vi "oa_SCL Draw XY Data.vi"(4 "[sized scatter plot cosmetics]":T1={"min size"=1, "max size"=5, "maps to max size"=5, "color array"=[16776960, 65280, 16711680, 255]}, 6 "xy cosmetics":T3={"plot color"=16776960, "plot type"=enum."connected points", "baseline"=0.0} {"baseline" format="%0.2f"}, 8 "xy data":cluster{"x":dbl, "y":dbl}[](array[cluster]) {"y" format="%0.2f"; "x" format="%0.2f"}, 9 "y scale factors":cluster{"a":dbl, "b":dbl, "log?":bool} {"b" format="%0.2f"; "a" format="%0.2f"}, 10 "x scale factors":cluster{"a":dbl, "b":dbl, "log?":bool} {"b" format="%0.2f"; "a" format="%0.2f"}, 11 "picture":picture) -> (3 "new picture":picture)   [LabVIEW 2017]
uses:
  <vilib>/picture/cartesn2.llb/XY Plot Type.ctl
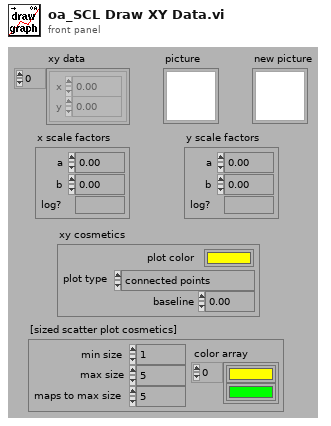
[diagram p1: front panel]
types:
  T1 = cluster{"min size":i16, "max size":i16, "maps to max size":i16, "color array":u32[]}
  T2 = typedef "XY Plot Type.ctl" = enum16{"points", "squares", "circles", "connected points", "connected squares", "connected circles", "comb plot", "sized scatter plot", "sized-colored scatter plot", "min-max lines"}
  T3 = cluster{"plot color":u32, "plot type":T2, "baseline":dbl}
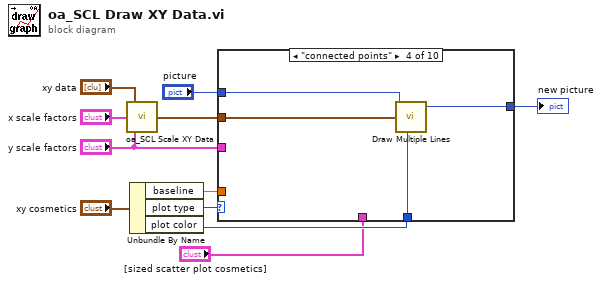
[diagram p0: block diagram]
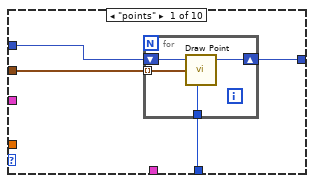
[diagram p2: hidden frame]
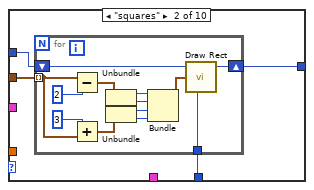
[diagram p3: hidden frame]
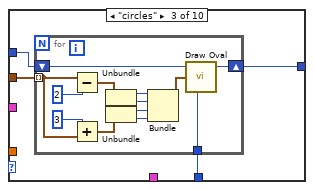
[diagram p4: hidden frame]
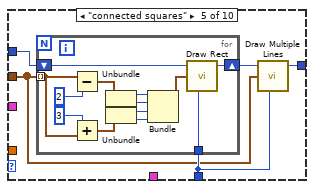
[diagram p5: hidden frame]
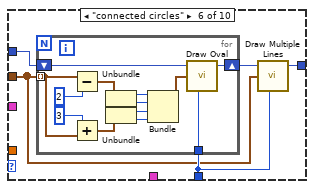
[diagram p6: hidden frame]
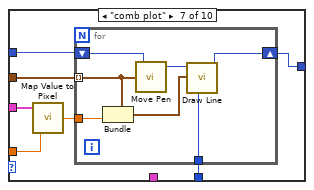
[diagram p7: hidden frame]
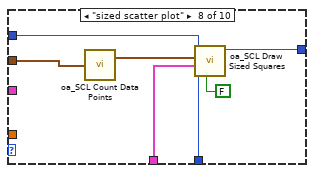
[diagram p8: hidden frame]
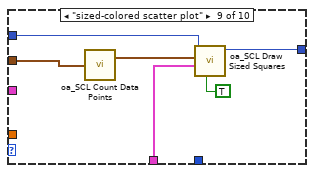
[diagram p9: hidden frame]
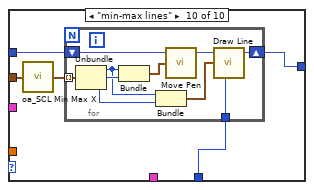
[diagram p10: hidden frame]
diagram:
  n1 = call <vilib>:"oa_SCL Scale XY Data.vi"("y scale factors"="y scale factors", "x scale factors"="x scale factors", "xy data"="xy data") -> ("scaled xy data"=w1:cluster{"x":i16, "y":i16}[])
  n2 = Unbundle By Name("xy cosmetics") -> ("baseline"=w4:dbl, "plot type"=w5:T2, "plot color"=w11:u32)
  n3 = case shown="\"connected points\"" w5 {
    tunnel: w11 -> [w15 w20 w37 w56 w62 w80 w94 w110 _ w124]
    tunnel: [w14 w21 w38 w57 w60 w78 w97 w114 w117 w121] -> w10
    tunnel: "picture" -> [w13 w22 w39 w54 w59 w77 w98 w111 w119 w125]
    tunnel: w1 -> [w12 w23 w40 w55 w58 w76 w96 w112 w120 w122]
    tunnel: w4 -> [_ _ _ _ _ _ w99 _ _ _]
    tunnel: "y scale factors" -> [_ _ _ _ _ _ w100 _ _ _]
    tunnel: "[sized scatter plot cosmetics]" -> [_ _ _ _ _ _ _ w109 w116 _]
    frame "points" {
      n4 = for {
        shift-right: [w19] -> w14
        shift-left: w13 -> [w18]
        tunnel: w15 -> [w17]
        tunnel: w12 -> [w16] mode=indexing
        n5 = call <vilib>:"Draw Point.vi"("picture"=w18, "point(x,y)"=w16, "color(black)"=w17) -> ("new picture"=w19:picture)  [unwired: 6 in]
      }
    }
    frame "squares" {
      n6 = for {
        tunnel: w23 -> [w33] mode=indexing
        shift-right: [w36] -> w21
        shift-left: w22 -> [w35]
        tunnel: w20 -> [w34]
        n7 = Subtract(x=w33, y=i16 2) -> (x-y=w26:cluster{"x":i16, "y":i16})
        n8 = Add(x=i16 3, y=w33) -> (x+y=w32:cluster{"x":i16, "y":i16})
        n9 = Unbundle(w26) -> ("x"=w28:i16, "y"=w29:i16)
        n10 = Unbundle(w32) -> ("x"=w30:i16, "y"=w31:i16)
        n11 = Bundle("x"=w28, "y"=w29, "x"=w30, "y"=w31) -> (w27:cluster{"x":i16, "y":i16, "x":i16, "y":i16})  [unwired: 1 in]
        n12 = call <vilib>:"Draw Rect.vi"("picture"=w35, "rect"=w27, "color(black)"=w34) -> ("new picture"=w36:picture)  [unwired: 6 in]
      }
    }
    frame "circles" {
      n13 = for {
        tunnel: w40 -> [w50] mode=indexing
        shift-right: [w53] -> w38
        shift-left: w39 -> [w52]
        tunnel: w37 -> [w51]
        n14 = Subtract(x=w50, y=i16 2) -> (x-y=w43:cluster{"x":i16, "y":i16})
        n15 = Add(x=i16 3, y=w50) -> (x+y=w49:cluster{"x":i16, "y":i16})
        n16 = Unbundle(w43) -> ("x"=w45:i16, "y"=w46:i16)
        n17 = Unbundle(w49) -> ("x"=w47:i16, "y"=w48:i16)
        n18 = Bundle("x"=w45, "y"=w46, "x"=w47, "y"=w48) -> (w44:cluster{"x":i16, "y":i16, "x":i16, "y":i16})  [unwired: 1 in]
        n19 = call <vilib>:"Draw Oval.vi"("picture"=w52, "rect"=w44, "color(black)"=w51) -> ("new picture"=w53:picture)  [unwired: 6 in]
      }
    }
    frame "connected points" {
      n20 = call <vilib>:"Draw Multiple Lines.vi"("picture"=w54, "line endpoints"=w55, "color(black)"=w56) -> ("new picture"=w57:picture)  [unwired: 6 in]
    }
    frame "connected squares" {
      n21 = for {
        tunnel: w58 -> [w66] mode=indexing
        shift-right: [w75] -> w61
        shift-left: w59 -> [w74]
        tunnel: w62 -> [w68]
        n22 = Subtract(x=w66, y=i16 2) -> (x-y=w65:cluster{"x":i16, "y":i16})
        n23 = Add(x=i16 3, y=w66) -> (x+y=w67:cluster{"x":i16, "y":i16})
        n24 = Unbundle(w65) -> ("x"=w73:i16, "y"=w72:i16)
        n25 = Unbundle(w67) -> ("x"=w71:i16, "y"=w70:i16)
        n26 = Bundle("x"=w73, "y"=w72, "x"=w71, "y"=w70) -> (w69:cluster{"x":i16, "y":i16, "x":i16, "y":i16})  [unwired: 1 in]
        n27 = call <vilib>:"Draw Rect.vi"("picture"=w74, "rect"=w69, "color(black)"=w68) -> ("new picture"=w75:picture)  [unwired: 6 in]
      }
      n28 = call <vilib>:"Draw Multiple Lines.vi"("picture"=w61, "line endpoints"=w58, "color(black)"=w62) -> ("new picture"=w60:picture)  [unwired: 6 in]
    }
    frame "connected circles" {
      n29 = for {
        tunnel: w76 -> [w84] mode=indexing
        shift-right: [w93] -> w79
        shift-left: w77 -> [w92]
        tunnel: w80 -> [w86]
        n30 = Subtract(x=w84, y=i16 2) -> (x-y=w83:cluster{"x":i16, "y":i16})
        n31 = Add(x=i16 3, y=w84) -> (x+y=w85:cluster{"x":i16, "y":i16})
        n32 = Unbundle(w83) -> ("x"=w91:i16, "y"=w90:i16)
        n33 = Unbundle(w85) -> ("x"=w89:i16, "y"=w88:i16)
        n34 = Bundle("x"=w91, "y"=w90, "x"=w89, "y"=w88) -> (w87:cluster{"x":i16, "y":i16, "x":i16, "y":i16})  [unwired: 1 in]
        n35 = call <vilib>:"Draw Oval.vi"("picture"=w92, "rect"=w87, "color(black)"=w86) -> ("new picture"=w93:picture)  [unwired: 6 in]
      }
      n36 = call <vilib>:"Draw Multiple Lines.vi"("picture"=w79, "line endpoints"=w76, "color(black)"=w80) -> ("new picture"=w78:picture)  [unwired: 6 in]
    }
    frame "comb plot" {
      n37 = call <vilib>:"Map Value to Pixel.vi"("x"=w99, "scale factors"=w100) -> ("pixel"=w95:dbl)  [unwired: 1 in]
      n38 = for {
        shift-right: [w105] -> w97
        shift-left: w98 -> [w107]
        tunnel: w96 -> [w103] mode=indexing
        tunnel: w95 -> [w104]
        tunnel: w94 -> [w101]
        n39 = Bundle(cluster=w103, "y"=w104) -> (w102:cluster{"x":i16, "y":i16})  [unwired: 1 in]
        n40 = call <vilib>:"Move Pen.vi"("new position"=w103, "picture"=w107) -> ("new picture"=w106:picture)  [unwired: 3 in]
        n41 = call <vilib>:"Draw Line.vi"("picture"=w106, "end point"=w102, "color(black)"=w101) -> ("new picture"=w105:picture)  [unwired: 6 in]
      }
    }
    frame "sized scatter plot" {
      n42 = call <vilib>:"oa_SCL Count Data Points.vi"("scaled xy data"=w112) -> ("counted data"=w113:cluster{"x":i16, "y":i16, "c":i16}[])  [unwired: 1 out]
      n43 = call <vilib>:"oa_SCL Draw Sized Squares.vi"("multi-color(F)"=FALSE, "color(yellow)"=w110, "sized scatter plot cosmetics"=w109, "data"=w113, "picture"=w111) -> ("new picture"=w114:picture)  [unwired: 6 in]
    }
    frame "sized-colored scatter plot" {
      n44 = call <vilib>:"oa_SCL Count Data Points.vi"("scaled xy data"=w120) -> ("counted data"=w118:cluster{"x":i16, "y":i16, "c":i16}[])  [unwired: 1 out]
      n45 = call <vilib>:"oa_SCL Draw Sized Squares.vi"("multi-color(F)"=TRUE, "sized scatter plot cosmetics"=w116, "data"=w118, "picture"=w119) -> ("new picture"=w117:picture)  [unwired: 7 in]
    }
    frame "min-max lines" {
      n46 = call <vilib>:"oa_SCL Min Max X.vi"("scaled xy data"=w122) -> ("min max data"=w123:cluster{"x":i16, "min":i16, "max":i16}[])
      n47 = for {
        shift-right: [w135] -> w121
        shift-left: w125 -> [w132]
        tunnel: w123 -> [w131] mode=indexing
        tunnel: w124 -> [w134]
        n48 = Unbundle(w131) -> ("x"=w127:i16, "min"=w129:i16, "max"=w128:i16)
        n49 = Bundle("x"=w127, "min"=w129) -> (w126:cluster{"x":i16, "min":i16})  [unwired: 1 in]
        n50 = Bundle("x"=w127, "max"=w128) -> (w130:cluster{"x":i16, "max":i16})  [unwired: 1 in]
        n51 = call <vilib>:"Move Pen.vi"("new position"=w126, "picture"=w132) -> ("new picture"=w133:picture)  [unwired: 3 in]
        n52 = call <vilib>:"Draw Line.vi"("picture"=w133, "end point"=w130, "color(black)"=w134) -> ("new picture"=w135:picture)  [unwired: 6 in]
      }
    }
  }
  "new picture" <- w10
